vi "Test Get Debug Data Log Contains Handled Data.vi"(8 "error in (no error)":errorcluster, 11 "Test Case In":refnum<class "Debugger Test.lvclass">) -> (0 "error out":errorcluster, 3 "Test Case Out":refnum<class "Debugger Test.lvclass">)   [LabVIEW 2020, in "Debugger Test.lvclass"]
uses:
  Debugger Test.lvclass
  C:/Program Files (x86)/National Instruments/LabVIEW 2020/vi.lib/Astemes/LUnit/Test Case.lvclass
  source/Debugger/Debugger.lvclass
  C:/Users/anton/Documents/GitHub/triarc-debugger/source/Process/Debug Process.lvclass
  source/Debug Data/Raw Debug Data.ctl
  source/Debug Data/Debug Data.lvclass/Debug Data.ctl
  source/Process/Debug Process.lvclass/Debug Process.ctl
  <vilib>/Astemes/LUnit/Test Case.lvclass/Test Case.ctl
  <vilib>/Astemes/LUnit/LUnit Assertion Result.lvclass/LUnit Assertion Result.ctl
  <vilib>/Astemes/LUnit/LUnit Test Case Result.lvclass/LUnit Test Case Result.ctl
  <vilib>/Astemes/LUnit/LUnit Method Result.lvclass/LUnit Method Result.ctl
  01074fa8-ee8a-411d-bc8b-fc92c4f90959.vi
  <vilib>/AdvancedString/Delimited String to 1D String Array.vi
  source/Process/Public/Lifecycle/Get Lifecycle State.vi
  source/Process/Private/SubVIs/Wait for finish.vi
  source/Process/Protected/Messaging/Enqueue Message.vi
  source/Process/Private/SubVIs/Set Lifecycle State.vi
  <vilib>/Astemes/LUnit/Palette/Pass.vi
  <vilib>/Astemes/LUnit/Palette/Fail.vi
  <vilib>/Astemes/LUnit/Compare Variants.vi
  <vilib>/Astemes/LUnit/Describe Comparison.vi
  <vilib>/Astemes/LUnit/Set Assertion Type.vi
  <vilib>/Utility/error.llb/Clear Errors.vi
  <vilib>/Astemes/LUnit/Add test result.vi
  <vilib>/Astemes/LUnit/LUnit Write Passed.vi
  <vilib>/Astemes/LUnit/LUnit Write Message.vi
  <vilib>/Astemes/LUnit/LUnit Write Description.vi
  <vilib>/Astemes/LUnit/Variant to string.vi
  <vilib>/Astemes/LUnit/LUnit Write Assertion Type.vi
  <vilib>/Astemes/LUnit/LUnit Record Assertion Result.vi
  <vilib>/Astemes/LUnit/LUnit Aggregate Assertion Results.vi
  <vilib>/Astemes/LUnit/Assertion Result/LUnit Read Status.vi
  <vilib>/Astemes/LUnit/LUnit Read Message.vi
  <vilib>/Astemes/LUnit/LUnit Read Description.vi
  <vilib>/Astemes/LUnit/Method Result/LUnit Merge Status.vi
  <vilib>/Astemes/LUnit/LUnit Concatenate result strings.vi
  <vilib>/Utility/error.llb/Error Cluster From Error Code.vi
  <vilib>/Utility/Data Type/Get Type Information.vi
  <vilib>/Utility/LVClass/Get LV Class Name.vi
  source/Debug Data/Debug Data.lvclass
  <vilib>/Astemes/LUnit/LUnit Assertion Result.lvclass
  source/Process/Debug Process.lvclass
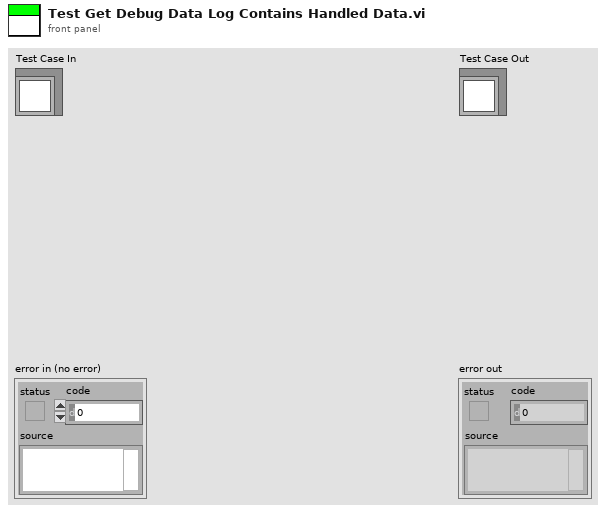
[diagram p1: front panel]
types:
  T1 = typedef "Debug Data.lvclass/Raw Debug Data.ctl" = cluster{"Action":string, "Call Chain":string, "Process":string, "Message":string, "Message Data":variant, "Time":dbl}
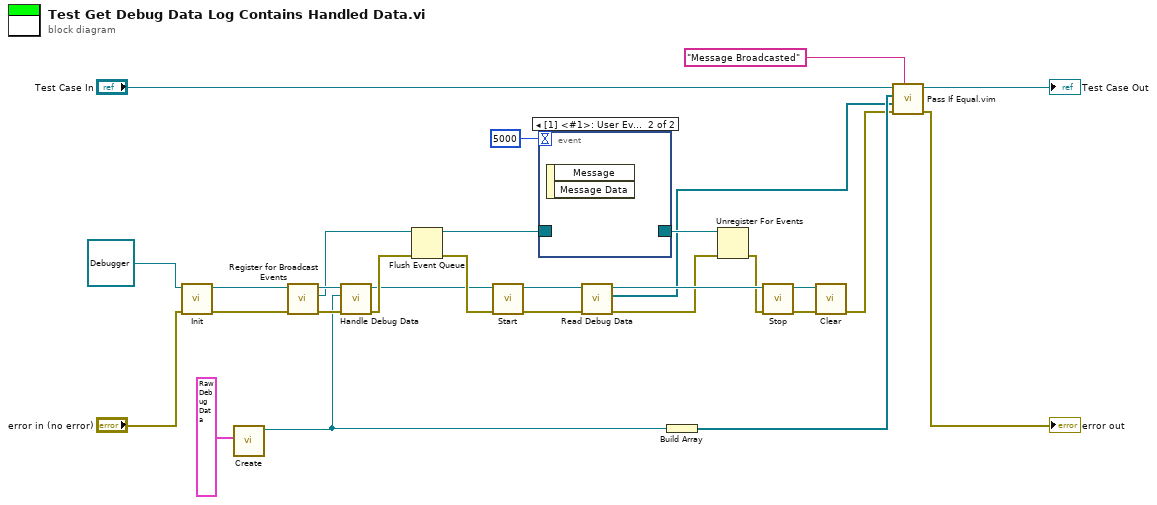
[diagram p0: block diagram]
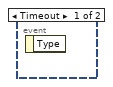
[diagram p2: hidden frame]
diagram:
  n1 = call-dynamic "Init.vi"("error in (no error)"="error in (no error)", "Process In"=refnum<class "Debugger.lvclass"> refnum ("Debug Data Event In 2")) -> ("error out"=w1:errorcluster, "Process Out"=w2:refnum<class "Debugger.lvclass">)  [unwired: 8 in]
  n2 = call "Create.vi"("Debug Data Cluster"=T1 {"Action"="", "Call Chain"="", "Process"="Test", "Message"="", "Message Data"=variant, "Time"=0.0}) -> ("Debug Data out"=w14:refnum<class "Debug Data.lvclass">)  [unwired: 9 in, 1 out]
  n3 = call "Register for Broadcast Events.vi"("error in (no error)"=w1, "Process In"=w2) -> ("error out"=w26:errorcluster, "Event Registration Refnum Out"=w11:refnum<event-registration>, "Process Out"=w21:refnum<class "Debugger.lvclass">)  [unwired: 7 in]
  n4 = call-dynamic "Handle Debug Data.vi"("error in (no error)"=w26, "Debug Data.lvclass"=w14, "Debug Data Event In"=w21) -> ("error out"=w25:errorcluster, "Debug Data Event Out"=w4:refnum<class "Debugger.lvclass">)  [unwired: 7 in]
  n5 = Flush Event Queue(0:w11, 3:w25) -> (8:w10:refnum<event-registration>, 11:w12:errorcluster)  [unwired: 4 in, 1 out]
  n6 = call "Start.vi"("error in (no error)"=w12, "Process In"=w4) -> ("error out"=w5:errorcluster, "Process Out"=w3:refnum<class "Debugger.lvclass">)  [unwired: 7 in, 1 out]
  n7 = event shown="[1] <#1>: User Event" {
    selector: w10 -> [_ _]
    dyn-events: [_ _] -> w16
    timeout: 5000 -> [_ _]
    event Timeout {
      n8 = event-data() -> ()  [unwired: 1 in, 1 out]
    }
    event User Event {
      n9 = event-data() -> ()  [unwired: 1 in, 2 out]
    }
  }
  n10 = call "Read Debug Data.vi"("error in (no error)"=w5, "Debugger In"=w3) -> ("error out"=w7:errorcluster, "Data Log"=w6:refnum<class "Debug Data.lvclass">[], "Debugger Out"=w24:refnum<class "Debugger.lvclass">)  [unwired: 7 in]
  n11 = Build Array(w14) -> (w13:refnum<class "Debug Data.lvclass">[])
  n12 = Unregister For Events(event registration refnum=w16, error in=w7) -> (error out=w8:errorcluster)
  n13 = call "Stop.vi"("error in (no error)"=w8, "Process In"=w24) -> ("error out"=w22:errorcluster, "Process Out"=w23:refnum<class "Debugger.lvclass">)  [unwired: 7 in, 1 out]
  n14 = call-dynamic "Clear.vi"("error in (no error)"=w22, "Process In"=w23) -> ("error out"=w9:errorcluster)  [unwired: 9 in]
  n15 = call "Pass If Equal.vim"("Description"="Message Broadcasted", "error in (no error)"=w9, "Actual"=w6, "Expected"=w13, "LUnit Test Case In"="Test Case In") -> ("error out"=→"error out":errorcluster, "LUnit Test Case Out"=→"Test Case Out":refnum<class "Debugger Test.lvclass">)  [unwired: 5 in]
